vi "GaseNamen ausgeben.vi"(8 "error in (no error)":errorcluster caption="Fehler (Eingang, kein Fehler)") -> (0 "error out":errorcluster caption="Fehler (Ausgang)", 1 "Komplettes Enum in String":string[][](array[string]), 2 "Vergleich":bool[](array[boolean]), 3 "GaseArray":string[](array[string]))   [LabVIEW 2020, in "Linearisierung v2.lvlib" / "Gasteiler.lvlib" / "HovaCal.lvlib"]
uses:
  HovaCal.lvlib
  Aktion_FGV_Betriebsdaten.ctl
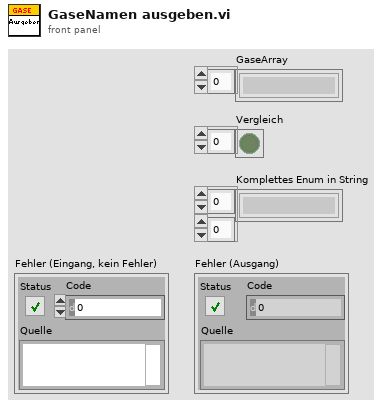
[diagram p1: front panel]
types:
  T1 = typedef "Linearisierung v2.lvlib/Gasteiler.lvlib/HovaCal.lvlib/Aktion_FGV_Betriebsdaten.ctl" = enum16{"Lesen", "Sollwerte schreiben", "Sollwerte lesen", "Gase schreiben", "Gase lesen", "Dynamische Werte", "GaseRef", "Gase aendern"}
  T2 = typedef "Linearisierung v2.lvlib/Gasteiler.lvlib/HovaCal.lvlib/Gase.ctl" = cluster{"Trägergas":u16, "Komponente 1":u16, "Komponente 2":u16}
  T3 = cluster{"Trägergas":bool, "Komponente 1":bool, "Komponente 2":bool}
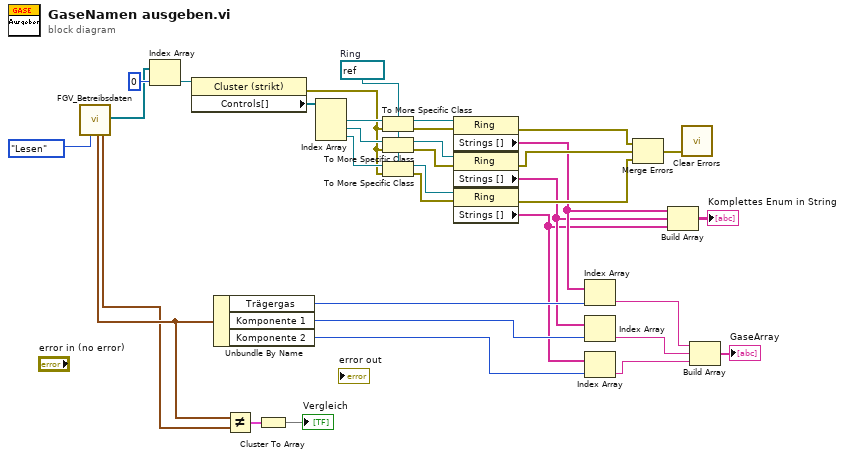
[diagram p0: block diagram]
diagram:
  w24 = refnum<vi> refnum  # Ring
  n1 = call "FGV_Betreibsdaten.vi"("Enum"=Aktion_FGV_Betriebsdaten."Lesen") -> ("Gase schreiben"=w27:T2, "Gase lesen"=w26:T2, "Array"=w30:refnum<vi>[])  [unwired: 11 in, 5 out]
  n2 = Index Array(array=w30, index=0 ("Index")) -> (element=w32:refnum<vi>)
  n3 = property class="Cluster (strikt)"(reference=w32) -> (error out=w9:errorcluster, "Controls[]"=w33:refnum<vi>[])  [unwired: 1 in, 1 out]
  n4 = Unbundle By Name(w27) -> ("Trägergas"=w16:u16, "Komponente 1"=w15:u16, "Komponente 2"=w14:u16)
  n5 = Not Equal?(x=w27, y=w26) -> (x != y?=w28:T3)
  n6 = Cluster To Array(cluster=w28) -> (array=→"Vergleich":bool[])
  n7 = Index Array(array=w33) -> (element #1=w34:refnum<vi>, element #2=w23:refnum<vi>, element #3=w22:refnum<vi>)  [unwired: 3 in]
  n8 = To More Specific Class(target class=w24, reference=w34, error in=w9) -> (specific class reference=w35:refnum<vi>, error out=w20:errorcluster)
  n9 = To More Specific Class(target class=w24, reference=w23, error in=w9) -> (specific class reference=w21:refnum<vi>, error out=w19:errorcluster)
  n10 = To More Specific Class(target class=w24, reference=w22, error in=w9) -> (specific class reference=w17:refnum<vi>, error out=w18:errorcluster)
  n11 = property class="Ring"(reference=w35, error in=w20) -> (error out=w8:errorcluster, "Strings []"=w4:string[])  [unwired: 1 out]
  n12 = property class="Ring"(reference=w21, error in=w19) -> (error out=w7:errorcluster, "Strings []"=w3:string[])  [unwired: 1 out]
  n13 = property class="Ring"(reference=w17, error in=w18) -> (error out=w6:errorcluster, "Strings []"=w2:string[])  [unwired: 1 out]
  n14 = Index Array(array=w4, index=w16) -> (element=w13:string)
  n15 = Index Array(array=w3, index=w15) -> (element=w12:string)
  n16 = Index Array(array=w2, index=w14) -> (element=w11:string)
  n17 = Merge Errors(w8, w7, w6) -> (w5:errorcluster)
  n18 = Build Array(w4, w3, w2) -> (→"Komplettes Enum in String":string[][])
  n19 = call <vilib>:"Clear Errors.vi"("error in (no error)"=w5) -> ()  [unwired: 5 in, 2 out]
  n20 = Build Array(w13, w12, w11) -> (→"GaseArray":string[])
